vi "测量数据区_选择.vi"(10 "Slave ID":u8=1, 11 "data":u16[](array[numeric]) format="%04xH") -> (3 "测量数据区":T1)   [LabVIEW 2016, in "斯坦道总磷总氮.lvlib"]
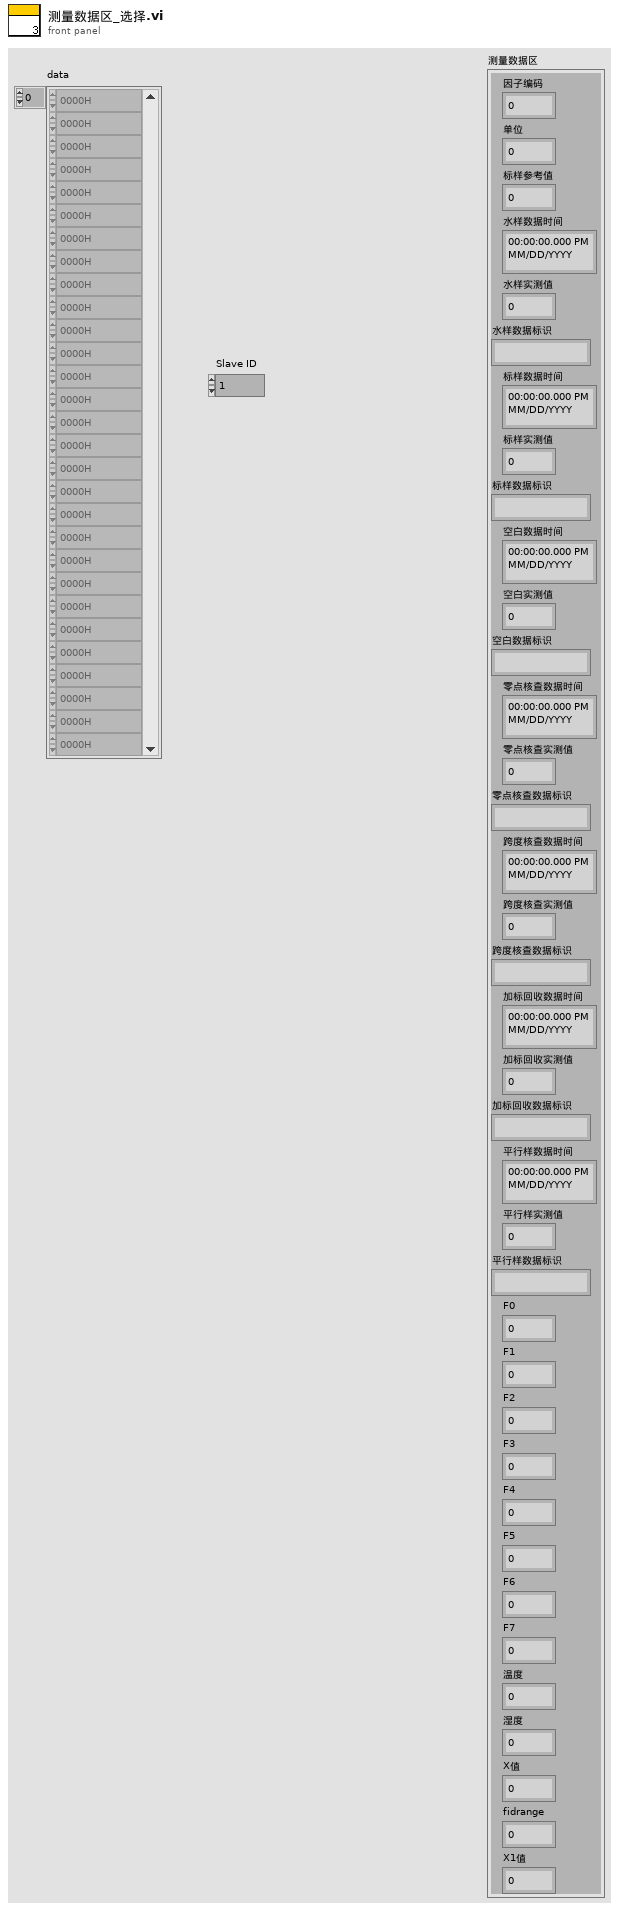
[diagram p1: front panel]
types:
  T1 = cluster{"因子编码":u32, "单位":u16, "标样参考值":sgl, "水样数据时间":timestamp, "水样实测值":sgl, "水样数据标识":string, "标样数据时间":timestamp, "标样实测值":sgl, "标样数据标识":string, "空白数据时间":timestamp, "空白实测值":sgl, "空白数据标识":string, "零点核查数据时间":timestamp, "零点核查实测值":sgl, "零点核查数据标识":string, "跨度核查数据时间":timestamp, "跨度核查实测值":sgl, "跨度核查数据标识":string, "加标回收数据时间":timestamp, "加标回收实测值":sgl, "加标回收数据标识":string, "平行样数据时间":timestamp, "平行样实测值":sgl, "平行样数据标识":string, "F0":sgl, "F1":sgl, "F2":sgl, "F3":sgl, "F4":sgl, "F5":sgl, "F6":sgl, "F7":sgl, "温度":sgl, "湿度":sgl, "X值":sgl, "fidrange":u16, "X1值":sgl}
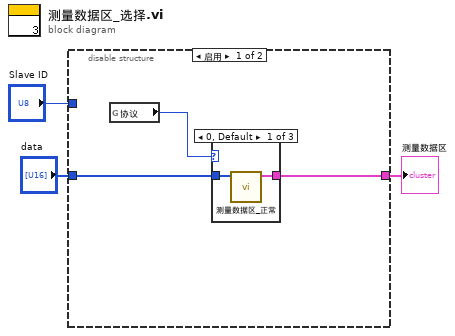
[diagram p0: block diagram]
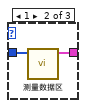
[diagram p2: hidden frame]
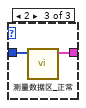
[diagram p3: hidden frame]
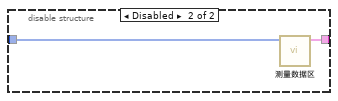
[diagram p4: hidden frame]
diagram:
  n1 = disable-structure shown="启用" {
    disable-tunnel: "Slave ID" -> [_ _]
    disable-tunnel: [w6 w13] -> w2
    disable-tunnel: "data" -> [w5 w14]
    frame Enabled {
      n2 = global read "总磷总氮断电保存全局变量.vi" "协议"() -> (w4:u16)
      n3 = case shown="0, Default" w4 {
        tunnel: w5 -> [w8 w10 w12]
        tunnel: [w7 w9 w11] -> w6
        frame 0, Default {
          n4 = call "测量数据区_正常.vi"("数组"=w8) -> ("测量数据区"=w7:T1)  [unwired: 10 in]
        }
        frame 1 {
          n5 = call "测量数据区.vi"("数组"=w10) -> ("测量数据区"=w9:T1)  [unwired: 10 in]
        }
        frame 2 {
          n6 = call "测量数据区_正常.vi"("数组"=w12) -> ("测量数据区"=w11:T1)  [unwired: 10 in]
        }
      }
    }
    frame Disabled {
      n7 = call "测量数据区.vi"("数组"=w14) -> ("测量数据区"=w13:T1)  [unwired: 10 in]
    }
  }
  "测量数据区" <- w2
